vi "AB_1200_1100_Project_Source_ExportedVI.vi"(7 "action":T3, 8 "error in (no error)":errorcluster, 9 "index in":i32, 10 "dataSource in":T1, 11 "buildObject":T2) -> (0 "error out":errorcluster, 1 "index out":i32, 2 "dataSource out":T1, 3 "buildObject out":T2)   [LabVIEW 2020]
doc: "Reads and writes the data to the object property bag."
uses:
  <resource>/Framework/Providers/API/ItemRef.ctl
  <vilib>/AppBuilder/RW_Project/AB_RW_Project_PropBag_Action.ctl
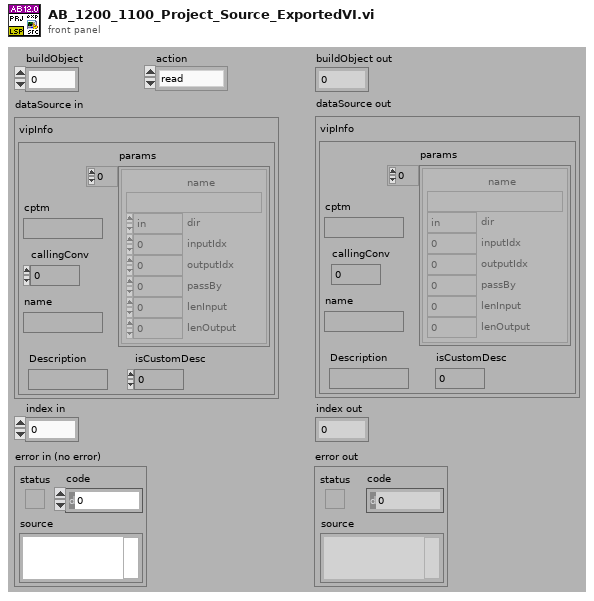
[diagram p1: front panel]
types:
  T1 = cluster{"vipInfo":cluster{"cptm":string, "params":cluster{"name":string, "dir":enum32{"in", "out", "in/out", "length", "error-out"}, "inputIdx":i32, "outputIdx":i32, "passBy":i32, "lenInput":i32, "lenOutput":i32}[], "callingConv":i32, "name":string, "Description":string, "isCustomDesc":i32}}
  T2 = typedef "ItemRef.ctl" = u64
  T3 = typedef "AB_RW_Project_PropBag_Action.ctl" = enum16{"read", "write", "clear", "readPrevious", "writePrevious", "clearPrevious"}
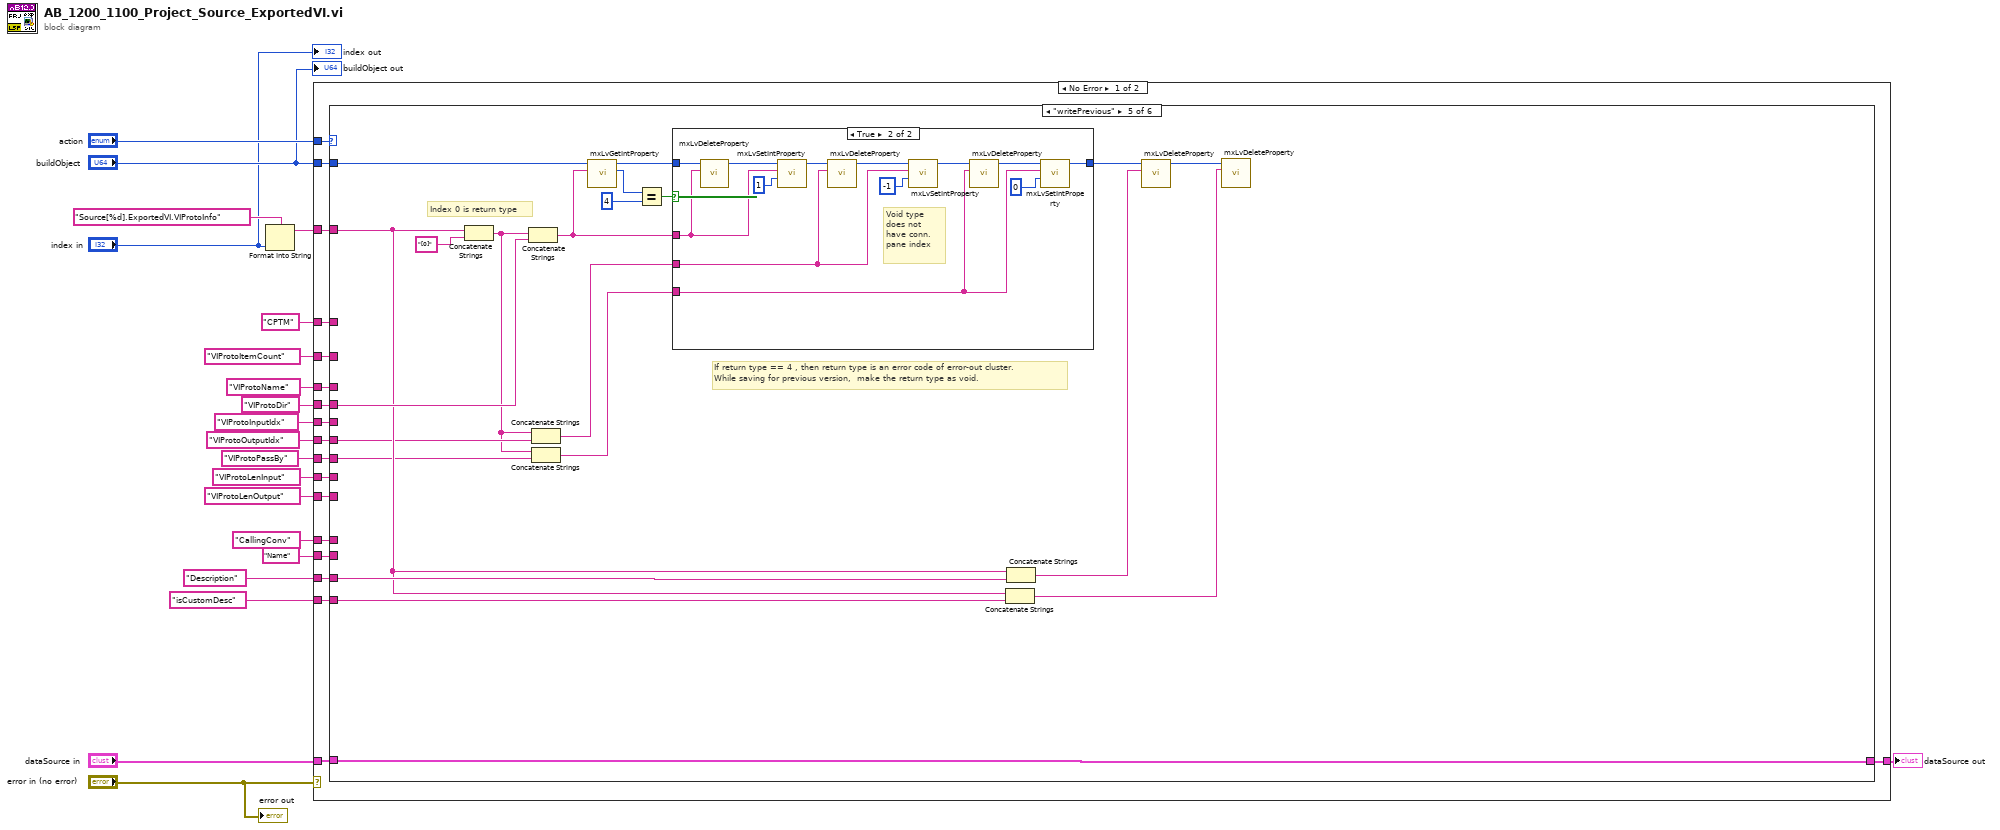
[diagram p0: block diagram]
diagram:
  n1 = Format Into String(format string="Source[%d].ExportedVI.VIProtoInfo", "index in") -> (resulting string=w19:string)  [unwired: 2 in, 1 out]
  n2 = case shown="No Error" "error in (no error)" {
    tunnel: "action" -> [w39 _]
    tunnel: "dataSource in" -> [w38 w80]
    tunnel: w19 -> [w37 _]
    tunnel: "buildObject" -> [w36 _]
    tunnel: [w35 w80] -> w14
    tunnel: "CPTM" -> [w34 _]
    tunnel: "VIProtoItemCount" -> [w33 _]
    tunnel: "VIProtoName" ("string") -> [w32 _]
    tunnel: "VIProtoDir" ("string") -> [w31 _]
    tunnel: "VIProtoInputIdx" ("string") -> [w30 _]
    tunnel: "VIProtoOutputIdx" ("string") -> [w29 _]
    tunnel: "VIProtoPassBy" ("string") -> [w28 _]
    tunnel: "VIProtoLenInput" ("string") -> [w27 _]
    tunnel: "VIProtoLenOutput" ("string") -> [w26 _]
    tunnel: "CallingConv" -> [w25 _]
    tunnel: "Name" -> [w24 _]
    tunnel: "Description" -> [w23 _]
    tunnel: "isCustomDesc" -> [w22 _]
    frame No Error {
      n3 = case shown="\"writePrevious\"" w39 {
        tunnel: w36 -> [_ _ _ _ w55 _]
        tunnel: w38 -> [w40 w41 w42 w43 w64 w79]
        tunnel: w37 -> [_ _ _ _ w56 _]
        tunnel: [w40 w41 w42 w43 w64 w79] -> w35
        tunnel: w34 -> [_ _ _ _ _ _]
        tunnel: w33 -> [_ _ _ _ _ _]
        tunnel: w32 -> [_ _ _ _ _ _]
        tunnel: w31 -> [_ _ _ _ w58 _]
        tunnel: w30 -> [_ _ _ _ _ _]
        tunnel: w29 -> [_ _ _ _ w47 _]
        tunnel: w28 -> [_ _ _ _ w48 _]
        tunnel: w27 -> [_ _ _ _ _ _]
        tunnel: w26 -> [_ _ _ _ _ _]
        tunnel: w25 -> [_ _ _ _ _ _]
        tunnel: w24 -> [_ _ _ _ _ _]
        tunnel: w23 -> [_ _ _ _ w63 _]
        tunnel: w22 -> [_ _ _ _ w62 _]
        frame "read" {
        }
        frame "write" {
        }
        frame "clear" {
        }
        frame "readPrevious" {
        }
        frame "writePrevious" {
          # "Index 0 is return type"
          # "If return type == 4 , then return type is an error code of error-out cluster.\nWhile saving for previous version,  make the return type as void."
          n4 = Concatenate Strings(w56, "[0]" ("string")) -> (w46:string)
          n5 = Concatenate Strings(w46, w58) -> (w49:string)
          n6 = Concatenate Strings(w46, w47) -> (w45:string)
          n7 = Concatenate Strings(w46, w48) -> (w44:string)
          n8 = call <resource>:"mxLvGetIntProperty.vi"("Tag"=w49, "Item"=w55) -> ("Value"=w54:i32, "Item"=w51:T2)  [unwired: 7 in, 1 out]
          n9 = Equal?(x=w54, y=4) -> (x = y?=w52:bool)
          n10 = case shown="True" w52 {
            tunnel: [w65 w68] -> w50
            tunnel: w51 -> [w65 w78]
            tunnel: w49 -> [_ w76]
            tunnel: w45 -> [_ w71]
            tunnel: w44 -> [_ w67]
            frame False {
            }
            frame True {
              # "Void type\ndoes not  \nhave conn.\npane index"
              n11 = call <resource>:"mxLvDeleteProperty.vi"("Tag"=w76, "Item"=w78) -> ("Item"=w77:T2)  [unwired: 8 in, 1 out]
              n12 = call <resource>:"mxLvSetIntProperty.vi"("Value (0)"=1, "Tag"=w76, "Item"=w77) -> ("Item"=w73:T2)  [unwired: 7 in, 1 out]
              n13 = call <resource>:"mxLvDeleteProperty.vi"("Tag"=w71, "Item"=w73) -> ("Item"=w72:T2)  [unwired: 8 in, 1 out]
              n14 = call <resource>:"mxLvSetIntProperty.vi"("Value (0)"=-1, "Tag"=w71, "Item"=w72) -> ("Item"=w69:T2)  [unwired: 7 in, 1 out]
              n15 = call <resource>:"mxLvDeleteProperty.vi"("Tag"=w67, "Item"=w69) -> ("Item"=w70:T2)  [unwired: 8 in, 1 out]
              n16 = call <resource>:"mxLvSetIntProperty.vi"("Value (0)"=0, "Tag"=w67, "Item"=w70) -> ("Item"=w68:T2)  [unwired: 7 in, 1 out]
            }
          }
          n17 = Concatenate Strings(w56, w62) -> (w59:string)
          n18 = Concatenate Strings(w56, w63) -> (w61:string)
          n19 = call <resource>:"mxLvDeleteProperty.vi"("Tag"=w61, "Item"=w50) -> ("Item"=w60:T2)  [unwired: 8 in, 1 out]
          n20 = call <resource>:"mxLvDeleteProperty.vi"("Tag"=w59, "Item"=w60) -> ()  [unwired: 8 in, 2 out]
        }
        frame "clearPrevious" {
        }
      }
    }
    frame Error {
    }
  }
  "dataSource out" <- w14
  "error out" <- "error in (no error)"
  "buildObject out" <- "buildObject"
  "index out" <- "index in"
